vi "Thermal Loop Test.vi"(8 "error in (no error)":errorcluster, 10 "Message IN":string) -> (0 "error out":errorcluster, 1 "Result (bool)":bool, 2 "Message OUT":string, 3 "VISA Refnum out":refnum<visa-resource-name>)   [LabVIEW 2022 SP3]
panel:
  in  "bypass":bool
  in  "stop":bool
  out "Instructional Message":string
  in  "OK Button":bool
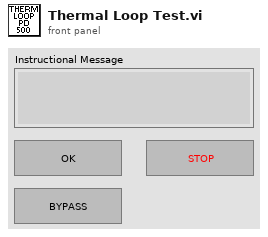
[diagram p1: front panel]
types:
  T1 = cluster{"Inst. Message":string, "Expected Filter Status":bool}[]
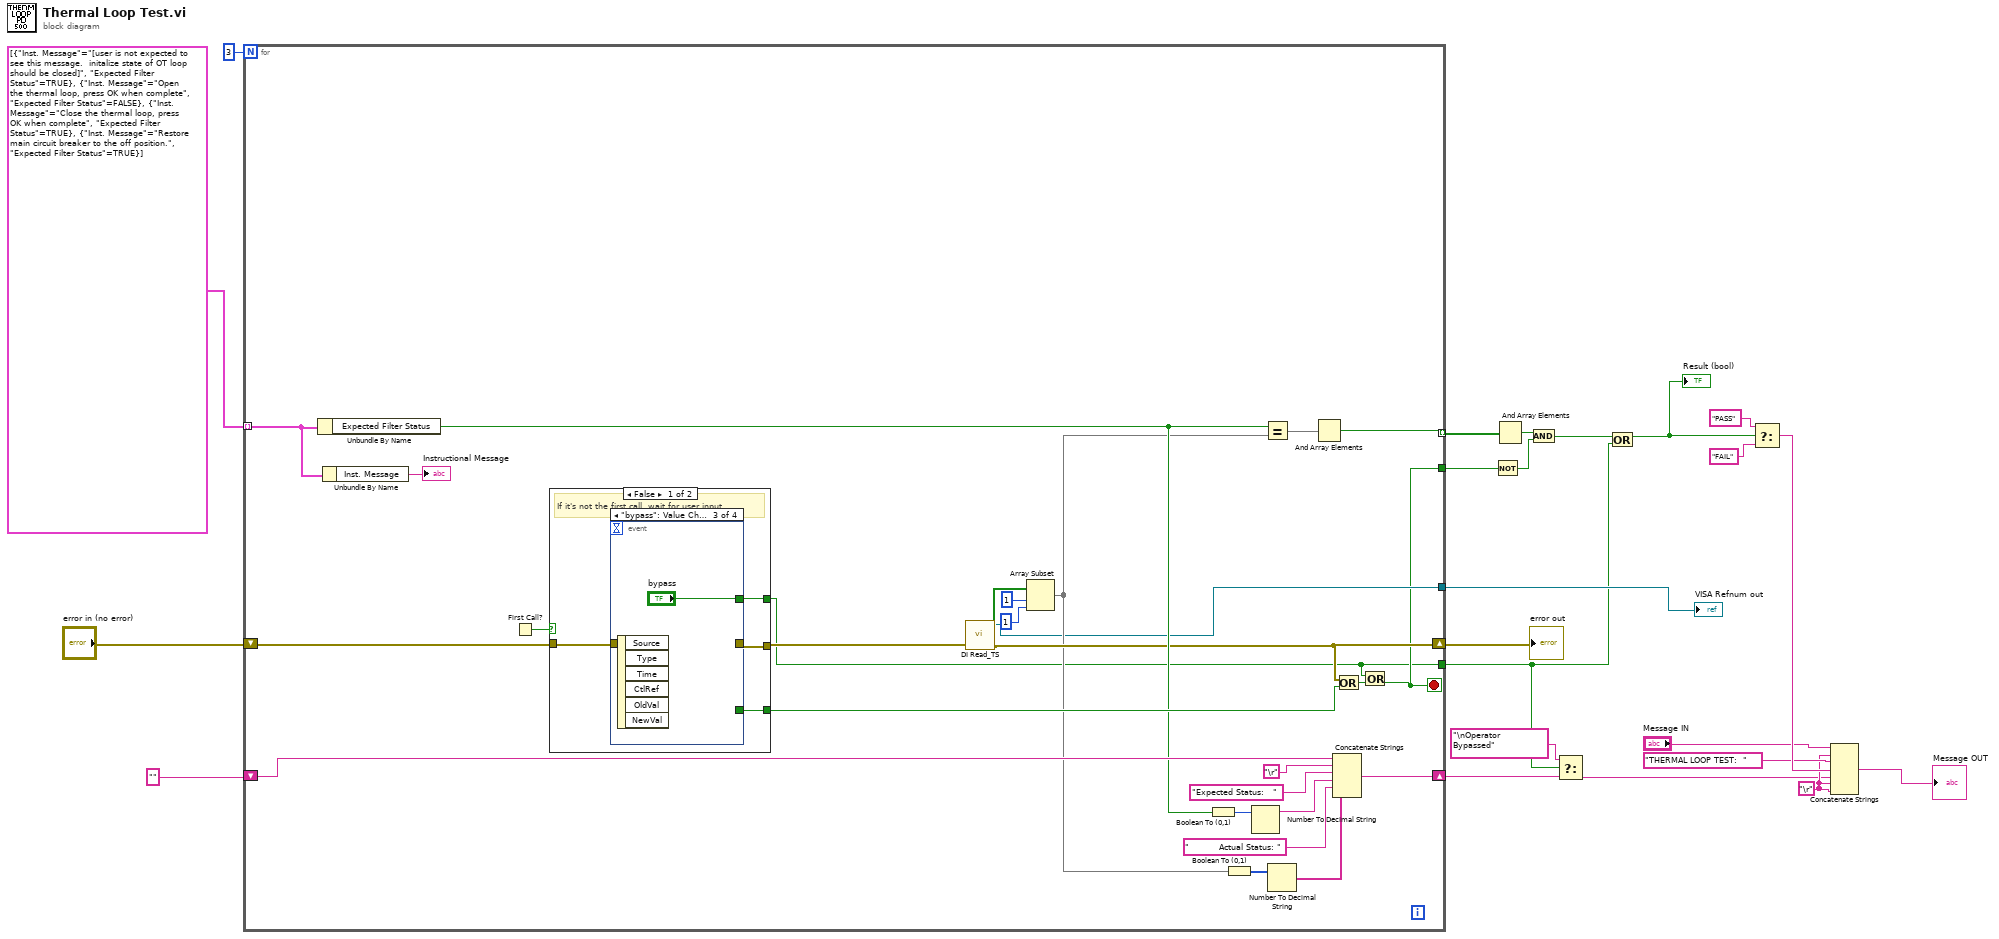
[diagram p0: block diagram]
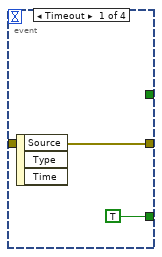
[diagram p2: hidden frame]
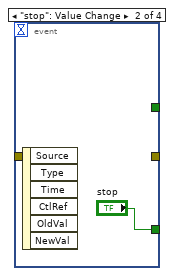
[diagram p3: hidden frame]
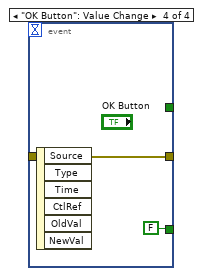
[diagram p4: hidden frame]
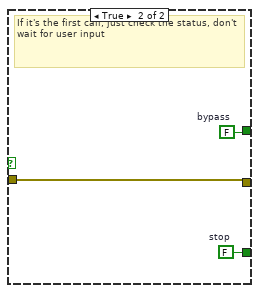
[diagram p5: hidden frame]
diagram:
  w13 = "\r"
  n1 = for {
    N: 3 -> [_]
    shift-right: [w29] -> w18
    shift-left: "error in (no error)" -> [w40]
    tunnel: [w36] -> w23 mode=indexing
    shift-right: [w43] -> w4
    shift-left: "" -> [w42]
    tunnel: T1 [{"Inst. Message"="[user is not expected to see this message.  initalize state of OT loop should be closed]", "Expected Filter Status"=TRUE}, {"Inst. Message"="Open the thermal loop, press OK when complete", "Expected Filter Status"=FALSE}, {"Inst. Message"="Close the thermal loop, press OK when complete", "Expected Filter Status"=TRUE}, {"Inst. Message"="Restore main circuit breaker to the off position.", "Expected Filter Status"=TRUE}] -> [w38] mode=indexing
    tunnel: [w25] -> w9
    tunnel: [w26] -> w6
    tunnel: [w24] -> w1
    stop <- w25 stop-if-true
    n2 = Unbundle By Name(w38) -> ("Expected Filter Status"=w34:bool)
    n3 = Unbundle By Name(w38) -> ("Inst. Message"=→"Instructional Message":string)
    n4 = First Call?() -> (First Call?: T/F=w27:bool)
    n5 = case shown="False" w27 {
      tunnel: w40 -> [w54 w63]
      tunnel: [w53 w62] -> w37
      tunnel: [w52 w63] -> w30
      tunnel: [w51 w61] -> w24
      frame False {
        # "If it's not the first call, wait for user input"
        n6 = event shown="[2] \"bypass\": Value Change" {
          selector: _ -> [_ _ _ _]
          dyn-events: _ -> [_ _ _ _]
          timeout: _ -> [_ _ _ _]
          tunnel: w54 -> [w56 _ _ w60]
          tunnel: [w56 _ _ w60] -> w52
          tunnel: [TRUE "stop" _ FALSE] -> w53
          tunnel: [_ _ "bypass" _] -> w51
          event Timeout {
            n7 = event-data() -> ()  [unwired: 1 in, 3 out]
          }
          event "stop": Value Change {
            n8 = event-data() -> ()  [unwired: 1 in, 6 out]
          }
          event "bypass": Value Change {
            n9 = event-data() -> ()  [unwired: 1 in, 6 out]
          }
          event "OK Button": Value Change {
            n10 = event-data() -> ()  [unwired: 1 in, 6 out]
          }
        }
      }
      frame True {
        w61 = FALSE  # bypass
        w62 = FALSE  # stop
        # "If it's the first call, just check the status, don't wait for user input"
      }
    }
    n11 = call "DI Read_TS.vi"("error in (no error)"=w30) -> ("error out"=w29:errorcluster, "DI Reading"=w33:bool[], "VISA Refnum out"=w26:refnum<visa-resource-name>)  [unwired: 7 in, 1 out]
    n12 = Array Subset(array=w33, index=1, length=1) -> (w28:bool[])
    n13 = Boolean To (0,1)(Boolean=w34) -> (0, 1=w45:i16)
    n14 = Boolean To (0,1)(Boolean=w28) -> (0, 1=w44:i16[])
    n15 = Number To Decimal String(number=w45) -> (decimal integer string=w48:string)  [unwired: 1 in]
    n16 = Equal?(x=w34, y=w28) -> (x = y?=w41:bool[])
    n17 = Number To Decimal String(number=w44) -> (decimal integer string=w50:string[])  [unwired: 1 in]
    n18 = And Array Elements(Boolean array=w41) -> (logical AND=w36:bool)
    n19 = Concatenate Strings(w42, "\r", "Expected Status:   ", w48, "          Actual Status: ", w50) -> (w43:string)
    n20 = Or(x=w29, y=w37) -> (x .or. y?=w35:bool)
    n21 = Or(x=w24, y=w35) -> (x .or. y?=w25:bool)
  }
  "error out" <- w18
  "VISA Refnum out" <- w6
  n22 = Not(x=w9) -> (.not. x?=w7:bool)
  n23 = And Array Elements(Boolean array=w23) -> (logical AND=w19:bool)
  n24 = And(x=w19, y=w7) -> (x .and. y?=w20:bool)
  n25 = Select(t="\nOperator Bypassed", s=w1, f=w4) -> (s? t:f=w5:string)
  n26 = Or(x=w20, y=w1) -> (x .or. y?=w2:bool)
  "Result (bool)" <- w2
  n27 = Select(t="PASS", s=w2, f="FAIL") -> (s? t:f=w16:string)
  n28 = Concatenate Strings("Message IN", w13, "THERMAL LOOP TEST:  ", w16, w5, w13, w13) -> (→"Message OUT":string)
